vi "Wait(ms) If Input Valid.vi"(8 "error in (no error)":errorcluster, 11 "milliseconds to wait(-1)":i32) -> (0 "error out":errorcluster)   [LabVIEW 2019, in "LabVIEW-ProviderShell.lvlib"]
uses:
  LabVIEW-ProviderShell.lvlib
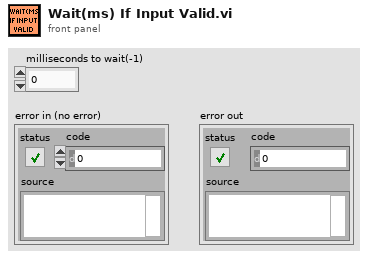
[diagram p1: front panel]
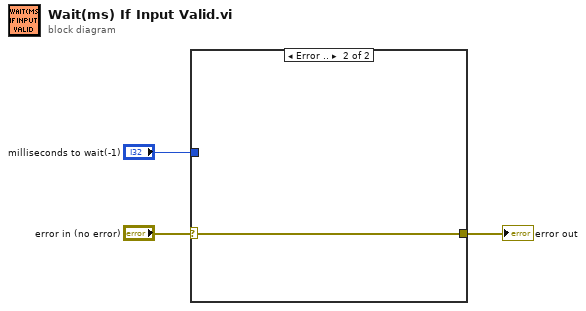
[diagram p0: block diagram]
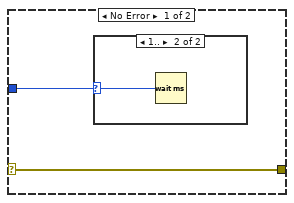
[diagram p2: hidden frame]
diagram:
  n1 = case shown="Error .." "error in (no error)" {
    selector: "error in (no error)" -> [w4 w7]
    tunnel: "milliseconds to wait(-1)" -> [w5 _]
    tunnel: [w4 w7] -> w1
    frame No Error {
      n2 = case shown="1.." w5 {
        selector: w5 -> [_ w6]
        frame 0, Default {
        }
        frame 1.. {
          n3 = Wait (ms)(milliseconds to wait=w6) -> ()  [unwired: 1 out]
        }
      }
    }
    frame Error {
    }
  }
  "error out" <- w1
